vi "Update Tree.vi"(8 "error in":errorcluster, 11 "state in":T1) -> (0 "error out":errorcluster, 3 "state out":T1)   [LabVIEW 2010, in "NI_SE_Config Front Panel Layout.lvlib"]
uses:
  NI_SE_Config Front Panel Layout.lvlib
  State.ctl
  VI Info.ctl
  VI Panel Layout/VI Panel Layout.lvclass
  VI Panel Layout/VI Panel Layout.lvclass/VI Panel Layout.ctl
  VI Panel Layout/Get VI Name.vi
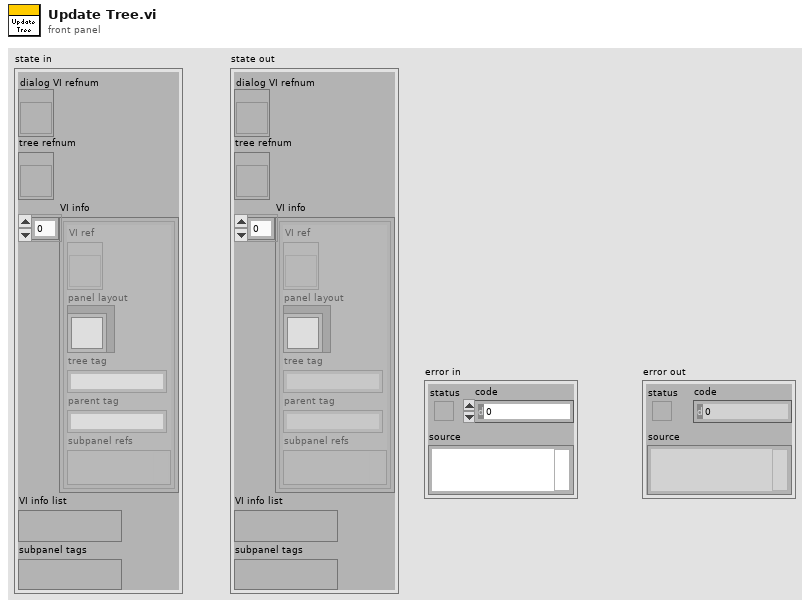
[diagram p1: front panel]
types:
  T1 = typedef "NI_SE_Config Front Panel Layout.lvlib/State.ctl" = cluster{"dialog VI refnum":refnum<vi>, "tree refnum":refnum<vi>, "VI info":T2[], "VI info list":variant, "subpanel tags":variant}
  T2 = typedef "NI_SE_Config Front Panel Layout.lvlib/VI Info.ctl" = cluster{"VI ref":refnum<vi>, "panel layout":refnum<class "VI Panel Layout.lvclass">, "tree tag":string, "parent tag":string, "subpanel refs":variant}
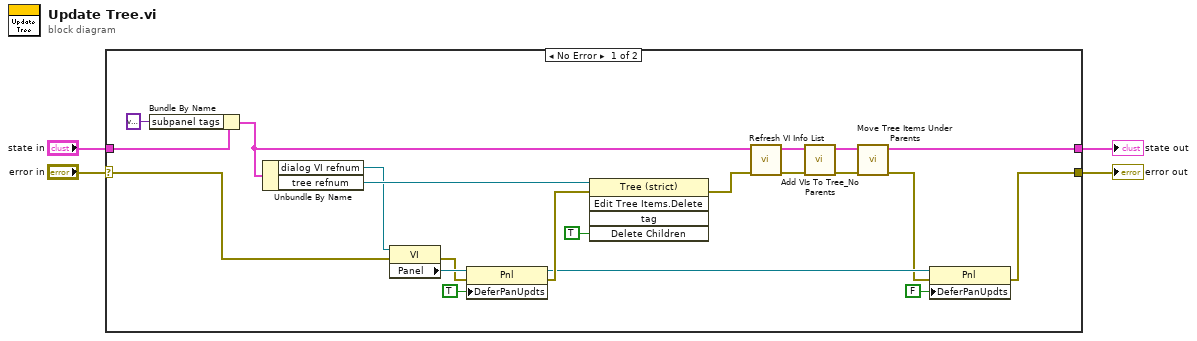
[diagram p0: block diagram]
diagram:
  n1 = case shown="No Error" "error in" {
    selector: "error in" -> [w16 w27]
    tunnel: "state in" -> [w23 w26]
    tunnel: [w9 w27] -> w2
    tunnel: [w19 w26] -> w1
    frame No Error {
      n2 = Bundle By Name(cluster=w23, "subpanel tags"=variant) -> (w8:T1)
      n3 = Unbundle By Name(w8) -> ("dialog VI refnum"=w17:refnum<vi>, "tree refnum"=w24:refnum<vi>)
      n4 = property class="VI"(reference=w17, error in=w16) -> (error out=w14:errorcluster, "Panel"=w18:refnum<vi>)  [unwired: 1 out]
      n5 = property class="Pnl"(reference=w18, error in=w14, "DeferPanUpdts"=TRUE ("Defer Panel Updates")) -> (reference out=w11:refnum<vi>, error out=w13:errorcluster)
      n6 = invoke class="Tree (strict)" method="Edit Tree Items.Delete"(reference=w24, error in=w13, "Delete Children"=TRUE ("Delete Children?")) -> (error out=w6:errorcluster)  [unwired: 2 in, 4 out]
      n7 = call "Refresh VI Info List.vi"("error in"=w6, "state in"=w8) -> ("error out"=w5:errorcluster, "state out"=w7:T1)  [unwired: 8 in]
      n8 = call "Add VIs To Tree_No Parents.vi"("error in"=w5, "state in"=w7) -> ("error out"=w20:errorcluster, "state out"=w21:T1)  [unwired: 8 in]
      n9 = call "Move Tree Items Under Parents.vi"("error in"=w20, "state in"=w21) -> ("error out"=w10:errorcluster, "state out"=w19:T1)  [unwired: 8 in]
      n10 = property class="Pnl"(reference=w11, error in=w10, "DeferPanUpdts"=FALSE ("Defer Panel Updates")) -> (error out=w9:errorcluster)  [unwired: 1 out]
    }
    frame Error {
    }
  }
  "state out" <- w1
  "error out" <- w2
